vi "Stop Nested Actors.vi"(8 "error in (no error)":errorcluster, 11 "Syringe in":refnum<class "Syringe Line.lvclass">) -> (0 "error out":errorcluster, 3 "Syringe out":refnum<class "Syringe Line.lvclass">)   [LabVIEW 2015, in "cRIO-Carbondioxide.lvlib" / "CO2-Actor.lvlib" / "Syringe Line.lvclass"]
uses:
  Syringe Line.lvclass
  Syringe Line.lvclass/Syringe Line.ctl
  <vilib>/ActorFramework/Message Enqueuer/Message Enqueuer.lvclass/Message Enqueuer.ctl
  <vilib>/ActorFramework/Message Enqueuer/Enqueue.vi
  <vilib>/ActorFramework/Message Priority Queue/Priority Enqueue.vi
  CO2 Actor/CO2 Actor.lvclass
  <vilib>/ActorFramework/Stop Msg/Stop Msg.lvclass
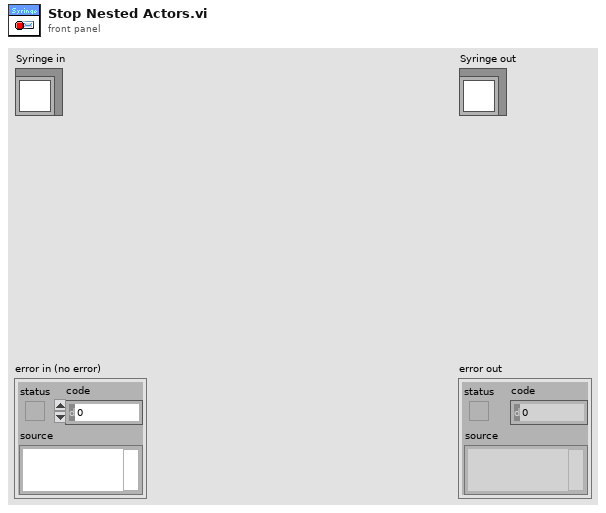
[diagram p1: front panel]
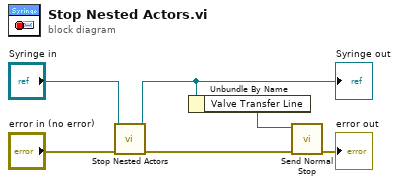
[diagram p0: block diagram]
diagram:
  n1 = call-parent "Stop Nested Actors.vi"("error in (no error)"="error in (no error)", "CO2 Actor in"="Syringe in") -> ("error out"=w4:errorcluster, "CO2 Actor out"=w1:refnum<class "Syringe Line.lvclass">)  [unwired: 8 in]
  "Syringe out" <- w1
  n2 = Unbundle By Name(w1) -> ("Valve Transfer Line"=w3:refnum<class "Message Enqueuer.lvclass">)
  n3 = call <vilib>:"Send Normal Stop.vi"("error in (no error)"=w4, "Message Enqueuer"=w3) -> ("error out"=→"error out":errorcluster)  [unwired: 9 in]
